vi "SPD.TR Bifurcation Meas Const T.vi"(4 "Temperature index":i32, 5 "Continue":refnum<vi>, 6 "deadtime index":i32, 7 "Progress":refnum<vi>, 8 "Error In":errorcluster, 11 "SPD.Stand Ctrl in":T1={"spdDeviceSession"={"spdRef"=0, "connected"=FALSE, "spdName"="", "specification"={"diod case"=enum."default", "type"=enum."Unknown", "frequency"=enum."Unknown"}, "hidSPD.Controller"={"TSet"=0.0, "HV_bias"=0.0, "DDS_stb_code"=0}, "hidSPD.Sturtup Values"={"TSet"=0.0, "HV_bias"=0.0, "DDS_stb_code"=0}}, "DevBSession"={"DevBRef"="", "connected"=FALSE}, "FreqCSession"={"FreqCRef"="", "timeout"=0.0, "Gate"=0.0, "connected"=FALSE}, "8164BSession"={"Connection ID"=refnum, "Connected"=FALSE, "Info"="", "Slots Info"=[]}, "LeCroySession"={"LeCroySession"="", "connected"=FALSE}, "Events"={"DCRTest"=refnum, "Stop"=refnum}, "configFile"={"configFile ref"=refnum, "configFile path"=path "", "equipmentFile ref"=refnum}, "SPD.Meas Grid"={"DateTime"="", "DT"=[], "Insensitivity"=[], "Temprature"=[], "Stb_code"=[], "HV_Bias"=[]}, "SPD.Queues"={"state queue"=refnum}, "Console"=refnum} {"spdDeviceSession"."hidSPD.Sturtup Values"."HV_bias" format="%#_6p, V"; "spdDeviceSession"."hidSPD.Sturtup Values"."TSet" format="%#_6p, DegC"; "spdDeviceSession"."hidSPD.Controller"."HV_bias" format="%#_6p, V"; "spdDeviceSession"."hidSPD.Controller"."TSet" format="%#_6p, DegC"}) -> (0 "Error Out":errorcluster, 1 "pass":bool, 2 "Report":string, 3 "SPD.Stand Ctrl out":T1={"spdDeviceSession"={"spdRef"=0, "connected"=FALSE, "spdName"="", "specification"={"diod case"=enum."default", "type"=enum."Unknown", "frequency"=enum."Unknown"}, "hidSPD.Controller"={"TSet"=0.0, "HV_bias"=0.0, "DDS_stb_code"=0}, "hidSPD.Sturtup Values"={"TSet"=0.0, "HV_bias"=0.0, "DDS_stb_code"=0}}, "DevBSession"={"DevBRef"="", "connected"=FALSE}, "FreqCSession"={"FreqCRef"="", "timeout"=0.0, "Gate"=0.0, "connected"=FALSE}, "8164BSession"={"Connection ID"=refnum, "Connected"=FALSE, "Info"="", "Slots Info"=[]}, "LeCroySession"={"LeCroySession"="", "connected"=FALSE}, "Events"={"DCRTest"=refnum, "Stop"=refnum}, "configFile"={"configFile ref"=refnum, "configFile path"=path "", "equipmentFile ref"=refnum}, "SPD.Meas Grid"={"DateTime"="", "DT"=[], "Insensitivity"=[], "Temprature"=[], "Stb_code"=[], "HV_Bias"=[]}, "SPD.Queues"={"state queue"=refnum}, "Console"=refnum} {"spdDeviceSession"."hidSPD.Sturtup Values"."HV_bias" format="%#_6p, V"; "spdDeviceSession"."hidSPD.Sturtup Values"."TSet" format="%#_6p, DegC"; "spdDeviceSession"."hidSPD.Controller"."HV_bias" format="%#_6p, V"; "spdDeviceSession"."hidSPD.Controller"."TSet" format="%#_6p, DegC"})   [LabVIEW 2018]
uses:
  typedefs/SPD.Stand Ctrl.ctl
  Instruments/SPD HID Interface/hidSPDLibForLabView/LibVIs/hidSPD Controls/hidSPD Device Session.ctl
  Instruments/SPD HID Interface/hidSPDLibForLabView/LibVIs/hidSPD Controls/hidSPD.SPD specification.ctl
  Instruments/SPD HID Interface/hidSPDLibForLabView/LibVIs/hidSPD Controls/hidSPD SPD Diod Case.ctl
  Instruments/SPD HID Interface/hidSPDLibForLabView/LibVIs/hidSPD Controls/hidSPD SPD Type.ctl
  Instruments/SPD HID Interface/hidSPDLibForLabView/LibVIs/hidSPD Controls/hidSPD.STB Frequency.ctl
  Instruments/SPD HID Interface/hidSPDLibForLabView/LibVIs/hidSPD Controls/hidSPD Controller.ctl
  Instruments/KC705 DevBoard/typedefs/DevB.Session.ctl
  Instruments/KeySight 53230A/typedefs/FreqC.Session.ctl
  Instruments/KeySight 8164B/KeySight 8164B LAN InstrLib/typedefs/KeySight 8164B control.ctl
  Instruments/LeCroy SDA830/typedefs/LeCroy.Session.ctl
  typedefs/SPD.Events.ctl
  ConfigFile/SPD.Config File ctrl.ctl
  <vilib>/Utility/config.llb/Config Data RefNum.ctl
  typedefs/SPD.Meas Grid.ctl
  typedefs/SPD.Queues.ctl
  typedefs/SPD.Stand state.ctl
  typedefs/SPD.Common HW Setup ctr.ctl
  typedefs/SPD.QE Strobe_Phase Tune Limits.ctl
  Instruments/KeySight 8164B/KeySight 8164B LAN InstrLib.lvlib
  <vilib>/Utility/config.llb/NI_LVConfig.lvlib
  Instruments/SPD HID Interface/hidSPDLibForLabView/hidSPDLibForLabView.lvlib
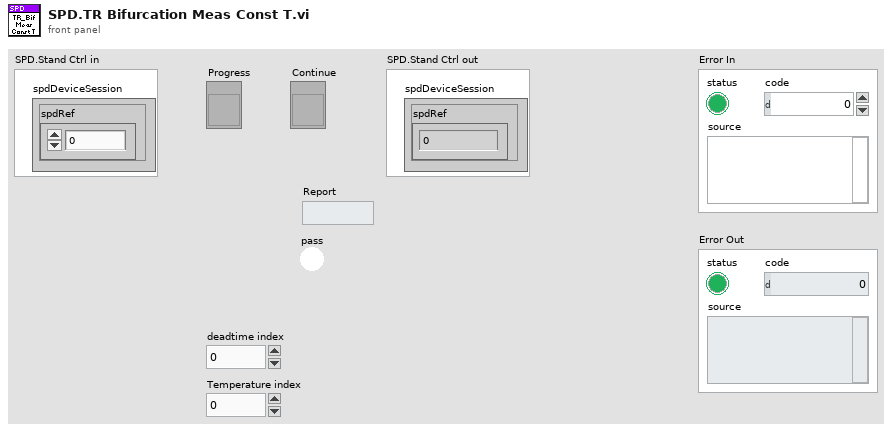
[diagram p1: front panel]
types:
  T1 = typedef "SPD.Stand Ctrl.ctl" = cluster{"spdDeviceSession":T2, "DevBSession":T8, "FreqCSession":T9, "8164BSession":T10, "LeCroySession":T11, "Events":T12, "configFile":T13, "SPD.Meas Grid":T15, "SPD.Queues":T16, "Console":refnum<vi>}
  T2 = typedef "hidSPDLibForLabView.lvlib/hidSPD Device Session.ctl" = cluster{"spdRef":u64, "connected":bool, "spdName":string, "specification":T3, "hidSPD.Controller":T7, "hidSPD.Sturtup Values":T7}
  T3 = typedef "hidSPDLibForLabView.lvlib/hidSPD.SPD specification.ctl" = cluster{"diod case":T4, "type":T5, "frequency":T6}
  T4 = typedef "hidSPDLibForLabView.lvlib/hidSPD SPD Diod Case.ctl" = enum16{"Unknown", "default", "butterfly"}
  T5 = typedef "hidSPDLibForLabView.lvlib/hidSPD SPD Type.ctl" = enum16{"Unknown", "Free Run", "Gate"}
  T6 = typedef "hidSPDLibForLabView.lvlib/hidSPD.STB Frequency.ctl" = enum16{"Unknown", "312", "1250"}
  T7 = typedef "hidSPDLibForLabView.lvlib/hidSPD Controller.ctl" = cluster{"TSet":sgl, "HV_bias":sgl, "DDS_stb_code":u16}
  T8 = typedef "DevB.Session.ctl" = cluster{"DevBRef":refnum<visa-resource-name>, "connected":bool}
  T9 = typedef "FreqC.Session.ctl" = cluster{"FreqCRef":refnum<visa-resource-name>, "timeout":dbl, "Gate":dbl, "connected":bool}
  T10 = typedef "KeySight 8164B LAN InstrLib.lvlib/KeySight 8164B control.ctl" = cluster{"Connection ID":refnum<k5>, "Connected":bool, "Info":string, "Slots Info":string[]}
  T11 = typedef "LeCroy.Session.ctl" = cluster{"LeCroySession":refnum<visa-resource-name>, "connected":bool}
  T12 = typedef "SPD.Events.ctl" = cluster{"DCRTest":refnum<user-event>, "Stop":refnum<user-event>}
  T13 = typedef "SPD.Config File ctrl.ctl" = cluster{"configFile ref":T14, "configFile path":path, "equipmentFile ref":T14}
  T14 = typedef "NI_LVConfig.lvlib/Config Data RefNum.ctl" = refnum<k1>
  T15 = typedef "SPD.Meas Grid.ctl" = cluster{"DateTime":string, "DT":dbl[], "Insensitivity":dbl[], "Temprature":dbl[], "Stb_code":dbl[], "HV_Bias":dbl[][][][]}
  T16 = typedef "SPD.Queues.ctl" = cluster{"state queue":refnum<queue>}
  T17 = typedef "SPD.Common HW Setup ctr.ctl" = cluster{"FS":i32, "TS":i32, "Gate":dbl, "Att1 enable":bool, "Att3 enable":bool, "Att3 Att":dbl, "Scope setup file path":string, "Pset":dbl, "Set Pset":bool}
  T18 = typedef "SPD.TR Test Params.ctl" = cluster{"FS":i32, "TS":i32, "Att3":dbl, "Pset_meas":dbl, "Pset_p_tune":dbl, "Gate":dbl, "Num of Meas":i32, "TRRecallFile":string, "TRHistoSize":i32, "Start index":i32}
  T19 = typedef "SPD.QE Strobe_Phase Tune Limits.ctl" = cluster{"ph_start":i32, "ph_stop":i32, "ph_step":i32}
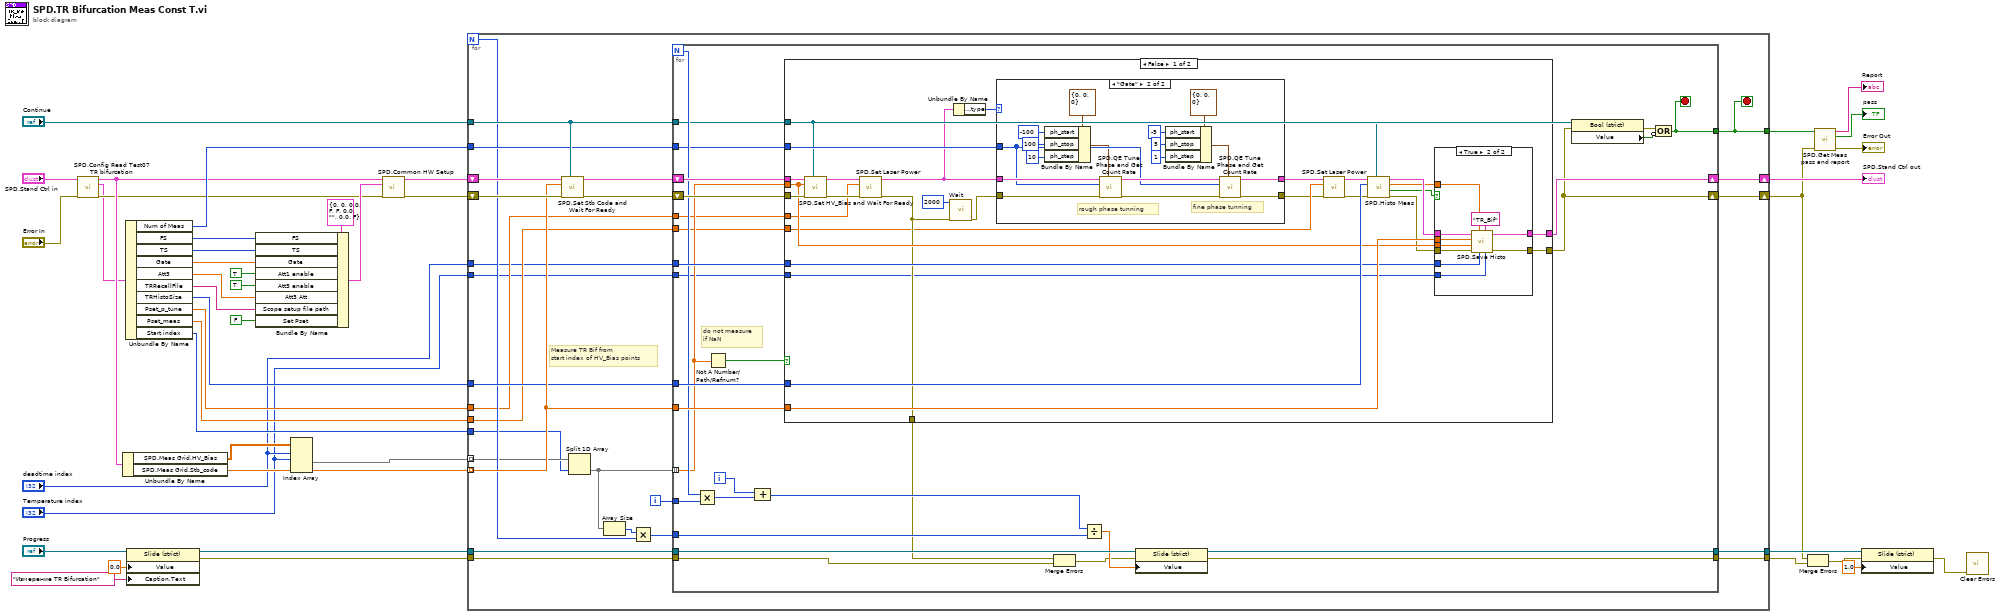
[diagram p0: block diagram]
diagram:
  n1 = call "SPD.Config Read Test07 TR bifurcation.vi"("Error In"="Error In", "SPD.Stand Ctrl in"="SPD.Stand Ctrl in") -> ("Error Out"=w15:errorcluster, "TR_Bif Meas Params"=w14:T18, "SPD.Stand Ctrl out"=w16:T1)  [unwired: 7 in]
  n2 = Unbundle By Name(w16) -> ("SPD.Meas Grid.HV_Bias"=w39:dbl[][][][], "SPD.Meas Grid.Stb_code"=w40:dbl[])
  n3 = Unbundle By Name(w14) -> ("Num of Meas"=w38:i32, "FS"=w24:i32, "TS"=w23:i32, "Gate"=w13:dbl, "Att3"=w12:dbl, "TRRecallFile"=w10:string, "TRHistoSize"=w11:i32, "Pset_p_tune"=w27:dbl, "Pset_meas"=w26:dbl, "Start index"=w28:i32)
  n4 = property class="Slide (strict)"(reference="Progress", "Value"=0.0, "Caption.Text"="Измерение TR Bifurcation") -> (reference out=w34:refnum<vi>, error out=w32:errorcluster)  [unwired: 1 in]
  n5 = Bundle By Name(cluster=T17 {"FS"=0, "TS"=0, "Gate"=0.0, "Att1 enable"=FALSE, "Att3 enable"=FALSE, "Att3 Att"=0.0, "Scope setup file path"="", "Pset"=0.0, "Set Pset"=FALSE} ("common hw setup"), "FS"=w24, "TS"=w23, "Gate"=w13, "Att1 enable"=TRUE, "Att3 enable"=TRUE, "Att3 Att"=w12, "Scope setup file path"=w10, "Set Pset"=FALSE) -> (w19:T17)
  n6 = Index Array(array=w39, index (dim 0)="deadtime index", index (dim 1)="Temperature index") -> (element=w36:dbl[][])  [unwired: 2 in]
  n7 = call "SPD.Common HW Setup.vi"("error in (no error)"=w15, "common hw setup"=w19, "SPD.Stand Ctrl in in"=w16) -> ("error out"=w8:errorcluster, "SPD.Stand Ctrl out"=w9:T1)  [unwired: 7 in]
  n8 = for {
    N -> [w55]
    tunnel: w36 -> [w52] mode=indexing
    tunnel: w40 -> [w62] mode=indexing
    shift-right: [w70] -> w37
    shift-left: w9 -> [w68]
    shift-right: [w69] -> w4
    shift-left: w8 -> [w67]
    tunnel: "Continue" -> [w60]
    tunnel: [w65] -> w5
    tunnel: w34 -> [w64]
    tunnel: [w63] -> w43
    tunnel: w38 -> [w59]
    tunnel: w11 -> [w61]
    tunnel: w32 -> [w54]
    tunnel: [w53] -> w30
    tunnel: w28 -> [w49]
    tunnel: w27 -> [w48]
    tunnel: w26 -> [w47]
    tunnel: "deadtime index" -> [w46]
    tunnel: "Temperature index" -> [w45]
    i -> [w66]
    stop <- w65 stop-if-true
    # "Measure TR Bif from\nstart index of HV_Bias points"
    n9 = call "SPD.Set Stb Code and Wait For Ready.vi"("Continue"=w60, "Error In"=w67, "Strobe code"=w62, "SPD.Stand Ctrl in"=w68) -> ("Error Out"=w57:errorcluster, "SPD.Stand Ctrl out"=w58:T1)  [unwired: 6 in]
    n10 = Split 1D Array(array=w52, index=w49) -> (second subarray=w51:dbl[])  [unwired: 1 out]
    n11 = Array Size(array=w51) -> (size(s)=w50:i32)
    n12 = Multiply(x=w50, y=w55) -> (x*y=w56:i32)
    n13 = for {
      N -> [w83]
      tunnel: w51 -> [w74] mode=indexing
      shift-right: [w86] -> w70
      shift-left: w58 -> [w100]
      shift-right: [w85] -> w69
      shift-left: w57 -> [w99]
      tunnel: w60 -> [w77]
      tunnel: w66 -> [w89]
      tunnel: [w96] -> w65
      tunnel: w64 -> [w95]
      tunnel: w56 -> [w93]
      tunnel: [w91] -> w63
      tunnel: w59 -> [w81]
      tunnel: w62 -> [w87]
      tunnel: w61 -> [w88]
      tunnel: w46 -> [w84]
      tunnel: w54 -> [w79]
      tunnel: [w78] -> w53
      tunnel: w48 -> [w73]
      tunnel: w47 -> [w72]
      tunnel: w45 -> [w71]
      i -> [w82]
      stop <- w96 stop-if-true
      # "do not measure\nif NaN"
      n14 = Multiply(x=w83, y=w89) -> (x*y=w90:i32)
      n15 = Not A Number/Path/Refnum?(number/path/refnum=w74) -> (NaN/Path/Refnum?=w75:bool)
      n16 = Compound Arithmetic op=ADD(w82, w90) -> (w94:i32)
      n17 = case shown="False" w75 {
        tunnel: w100 -> [w128 w161]
        tunnel: w99 -> [w127 w160]
        tunnel: w88 -> [w126 _]
        tunnel: w87 -> [w125 _]
        tunnel: w74 -> [w124 _]
        tunnel: [w123 w161] -> w86
        tunnel: [w122 w160] -> w85
        tunnel: w84 -> [w121 _]
        tunnel: w81 -> [w117 _]
        tunnel: w77 -> [w115 _]
        tunnel: [w108 w160] -> w76
        tunnel: w73 -> [w107 _]
        tunnel: w72 -> [w106 _]
        tunnel: w71 -> [w101 _]
        frame False {
          n18 = call "SPD.Set HV_Bias and Wait For Ready.vi"("Continue"=w115, "Error In"=w127, "HV_Bias"=w124, "SPD.Stand Ctrl in"=w128) -> ("Error Out"=w110:errorcluster, "SPD.Stand Ctrl out"=w111:T1)  [unwired: 6 in]
          n19 = call "SPD.Set Laser Power.vi"("Error In"=w110, "Pset"=w107, "SPD.Stand Ctrl in"=w111) -> ("Error Out"=w108:errorcluster, "SPD.Stand Ctrl out"=w109:T1)  [unwired: 7 in]
          n20 = call "Wait.vi"("error in (no error)"=w108, "milliseconds to wait"=u32 2000) -> ("error out"=w113:errorcluster)  [unwired: 9 in]
          n21 = Unbundle By Name(w109) -> ("spdDeviceSession.specification.type"=w116:T5)
          n22 = case shown="\"Gate\"" w116 {
            tunnel: [w130 w142] -> w105
            tunnel: [w129 w141] -> w104
            tunnel: w109 -> [w130 w140]
            tunnel: w117 -> [_ w133]
            tunnel: w113 -> [w129 w131]
            frame "Free Run", Default {
            }
            frame "Gate" {
              # "fine phase tunning"
              # "rough phase tunning"
              n23 = Bundle By Name(cluster=T19 {"ph_start"=0, "ph_stop"=0, "ph_step"=0} ("SPD.QE Strobe_Phase Tune Limits"), "ph_start"=-100, "ph_stop"=100, "ph_step"=10) -> (w132:T19)
              n24 = call "SPD.QE Tune Phase and Get Count Rate.vi"("SPD.QE Strobe_Phase Tune Limits"=w132, "Error In"=w131, "Num of FreqC Meas"=w133, "SPD.Stand Ctrl in"=w140) -> ("Error Out"=w138:errorcluster, "SPD.Stand Ctrl out"=w139:T1)  [unwired: 4 in, 2 out]
              n25 = Bundle By Name(cluster=T19 {"ph_start"=0, "ph_stop"=0, "ph_step"=0} ("SPD.QE Strobe_Phase Tune Limits"), "ph_start"=-5, "ph_stop"=5, "ph_step"=1) -> (w146:T19)
              n26 = call "SPD.QE Tune Phase and Get Count Rate.vi"("SPD.QE Strobe_Phase Tune Limits"=w146, "Error In"=w138, "Num of FreqC Meas"=w133, "SPD.Stand Ctrl in"=w139) -> ("Error Out"=w141:errorcluster, "SPD.Stand Ctrl out"=w142:T1)  [unwired: 4 in, 2 out]
            }
          }
          n27 = call "SPD.Set Laser Power.vi"("Error In"=w104, "Pset"=w106, "SPD.Stand Ctrl in"=w105) -> ("Error Out"=w102:errorcluster, "SPD.Stand Ctrl out"=w103:T1)  [unwired: 7 in]
          n28 = call "SPD.Histo Meas.vi"("Continue"=w115, "Error In"=w102, "Histo length"=w126, "SPD.Stand Ctrl in"=w103) -> ("Error Out"=w118:errorcluster, "pass"=w114:bool, "Histo"=w119:dbl[], "SPD.Stand Ctrl out"=w120:T1)  [unwired: 4 in]
          n29 = case shown="True" w114 {
            tunnel: w125 -> [_ w159]
            tunnel: w124 -> [_ w158]
            tunnel: [w149 w157] -> w123
            tunnel: [w148 w156] -> w122
            tunnel: w121 -> [_ w155]
            tunnel: w120 -> [w149 w154]
            tunnel: w119 -> [_ w153]
            tunnel: w118 -> [w148 w152]
            tunnel: w101 -> [_ w150]
            frame False {
            }
            frame True {
              n30 = call "SPD.Save Histo.vi"("Temperature index"=w150, "Name"="TR_Bif", "DT index"=w155, "AP Histo"=w153, "Error In"=w152, "HV_bias"=w158, "Stb_Code"=w159, "SPD.Stand Ctrl in"=w154) -> ("Error Out"=w156:errorcluster, "SPD.Stand Ctrl out"=w157:T1)  [unwired: 2 in]
            }
          }
        }
        frame True {
        }
      }
      n31 = Merge Errors(w76, w79) -> (w80:errorcluster)
      n32 = Divide(x=w94, y=w93) -> (x/y=w92:dbl)
      n33 = property class="Slide (strict)"(reference=w95, error in=w80, "Value"=w92) -> (reference out=w91:refnum<vi>, error out=w78:errorcluster)
      n34 = property class="Bool (strict)"(reference=w77, error in=w85) -> (error out=w97:errorcluster, "Value"=w98:bool)  [unwired: 1 out]
      n35 = Compound Arithmetic op=OR(w97, invert w98) -> (w96:bool)
    }
  }
  "SPD.Stand Ctrl out" <- w37
  n36 = Merge Errors(w4, w30) -> (w31:errorcluster)
  n37 = call "SPD.Get Meas pass and report.vi"("error in (no error)"=w4, "error or stoped"=w5) -> ("error out"=→"Error Out":errorcluster, "pass"=→"pass":bool, "report"=→"Report":string)  [unwired: 7 in]
  n38 = property class="Slide (strict)"(reference=w43, error in=w31, "Value"=1.0) -> (error out=w41:errorcluster)  [unwired: 1 out]
  n39 = call <vilib>:"Clear Errors.vi"("error in (no error)"=w41) -> ()  [unwired: 5 in, 2 out]
